vi "Stop Core Wrapper.vi"(10 "final error code in":i32, 11 "Controller in":refnum<class "Controller.lvclass">) -> (2 "final error code out":i32, 3 "Controller out":refnum<class "Controller.lvclass">)   [LabVIEW 2014, in "Controller.lvlib" / "Controller.lvclass"]
uses:
  Controller/Controller.lvclass
  SuperActor/Ex Nested.lvclass/Ex Nested.ctl
  Controller/Controller.lvclass/Controller.ctl
  reusable/Switch/Switch.lvclass
  SuperActor/Read Log Session.vi
  <userlib>/_Session Fwk/Session - Root.lvclass
  reusable/Session APIs/Session Log/System Log.lvclass
  <vilib>/NI_Real-Time Target Support.lvlib
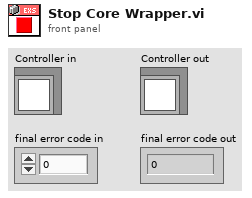
[diagram p1: front panel]
types:
  T1 = typedef "Session - Root.lvclass/Session Handle.ctl" = refnum<data-value>
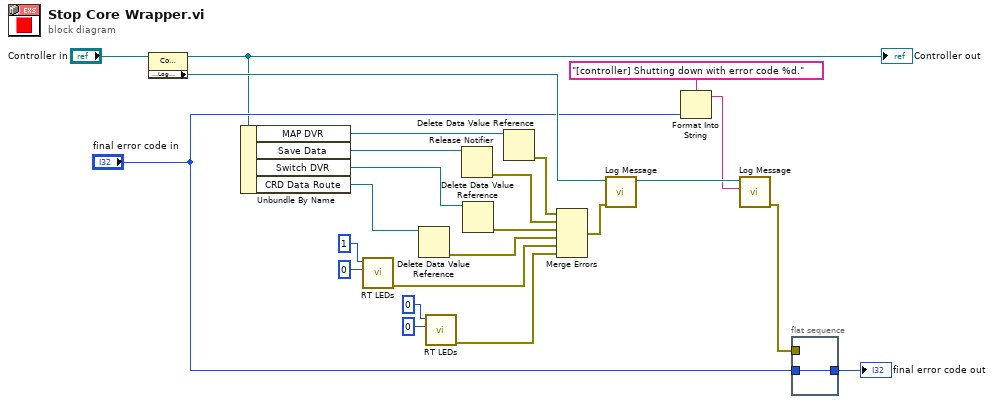
[diagram p0: block diagram]
diagram:
  n1 = property class="Controller"(reference="Controller in") -> (reference out=w1:refnum<class "Controller.lvclass">, "Accessors:Log Session"=w23:T1)  [unwired: 1 in, 1 out]
  "Controller out" <- w1
  n2 = Unbundle By Name(w1) -> ("MAP DVR"=w24:refnum<data-value>, "Save Data"=w2:refnum<notifier>, "Switch DVR"=w7:refnum<data-value>, "CRD Data Route"=w10:refnum<data-value>)
  n3 = call <vilib>:"RT LEDs.vi"("State"=0 ("LED Num"), "LED Num"=1) -> ("error out"=w15:errorcluster)  [unwired: 4 in, 1 out]
  n4 = Delete Data Value Reference(data value reference=w10) -> (error out=w16:errorcluster)  [unwired: 1 in, 1 out]
  n5 = call <vilib>:"RT LEDs.vi"("State"=0, "LED Num"=0) -> ("error out"=w14:errorcluster)  [unwired: 4 in, 1 out]
  n6 = Release Notifier(notifier=w2) -> (error out=w12:errorcluster)  [unwired: 2 in, 2 out]
  n7 = Delete Data Value Reference(data value reference=w7) -> (error out=w13:errorcluster)  [unwired: 1 in, 1 out]
  n8 = Delete Data Value Reference(data value reference=w24) -> (error out=w11:errorcluster)  [unwired: 1 in, 1 out]
  n9 = Merge Errors(w11, w12, w13, w16, w15, w14) -> (w17:errorcluster)
  n10 = call "Log Message.vi"("error in"=w17, "session in"=w23) -> ("session out"=w18:T1)  [unwired: 8 in, 1 out]
  n11 = Format Into String(format string="[controller] Shutting down with error code %d.", "final error code in") -> (resulting string=w4:string)  [unwired: 2 in, 1 out]
  n12 = call "Log Message.vi"("MSG In"=w4, "session in"=w18) -> ("error out"=w19:errorcluster)  [unwired: 8 in, 1 out]
  n13 = flat-sequence {
    tunnel: "final error code in" -> [w25]
    tunnel: w19 -> [_]
    tunnel: [w25] -> w21
    frame #0 {
    }
  }
  "final error code out" <- w21
